vi "Handle Request.vi"(7 "Processing In":refnum<class "Processing.lvclass">, 11 "HTTPStatsHandler in":refnum<class "HTTPStatsHandler.lvclass">) -> (0 "error out":errorcluster, 5 "Processing":refnum<class "Processing.lvclass">)   [LabVIEW 2020, in "Vecto.lvlib" / "HTTPStatsHandler.lvclass"]
uses:
  HTTPStatsHandler.lvclass
  <vilib>/IlluminatedG/IG HTTP Server/HTTP Server/Processing/Processing.lvclass
  HTTPStatsHandler.lvclass/HTTPStatsHandler.ctl
  VectoService/VectoService.lvclass
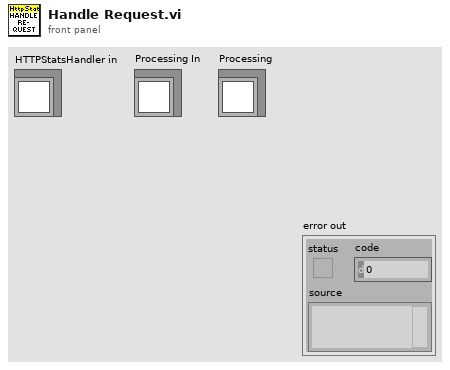
[diagram p1: front panel]
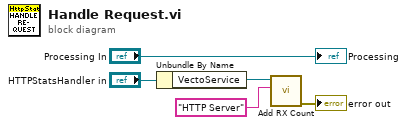
[diagram p0: block diagram]
diagram:
  n1 = Unbundle By Name("HTTPStatsHandler in") -> ("VectoService"=w1:refnum<class "VectoService.lvclass">)
  n2 = call "Add RX Count.vi"("Connection Name"="HTTP Server", "VectoService in"=w1) -> ("error out"=→"error out":errorcluster)  [unwired: 8 in, 1 out]
  "Processing" <- "Processing In"
